vi "Decorate.vi"(8 "error in (no error)":errorcluster, 10 "Decorator":refnum<class "uPolicy.lvclass">, 11 "Decorate in":refnum<class "Decorate.lvclass">) -> (0 "error out":errorcluster, 3 "Decorate out":refnum<class "Decorate.lvclass">)   [LabVIEW 2023, in "uLib.lvlib" / "Decorate.lvclass"]
doc: "Append a subscription policy, expand the property node to append multiple policies."
uses:
  Decorate.lvclass
  uPolicy/uPolicy.lvclass
  Decorate.lvclass/Decorate.ctl
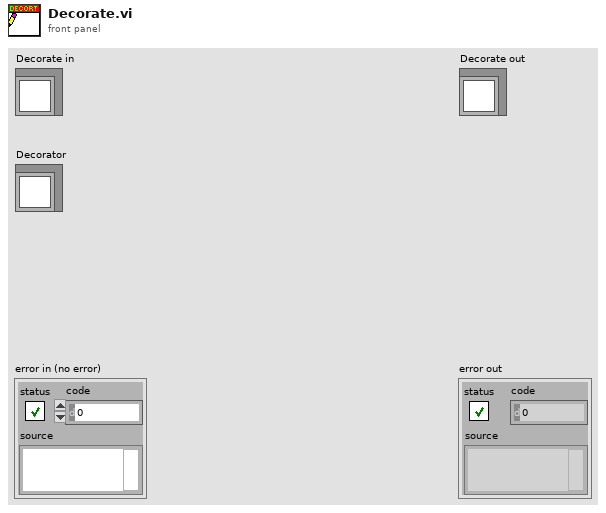
[diagram p1: front panel]
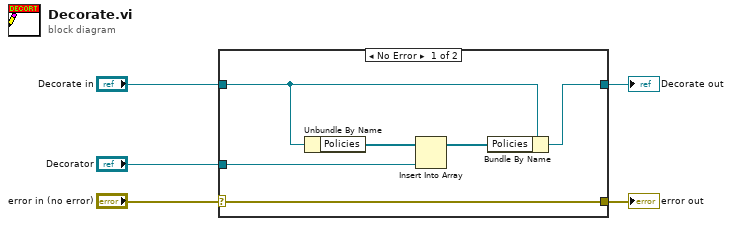
[diagram p0: block diagram]
diagram:
  n1 = case shown="No Error" "error in (no error)" {
    selector: "error in (no error)" -> [w11 w12]
    tunnel: [w11 w12] -> w4
    tunnel: [w10 w13] -> w2
    tunnel: "Decorate in" -> [w9 w13]
    tunnel: "Decorator" -> [w6 _]
    frame No Error {
      n2 = Unbundle By Name(w9) -> ("Policies"=w8:refnum<class "uPolicy.lvclass">[])
      n3 = Insert Into Array(array=w8, new element=w6) -> (w7:refnum<class "uPolicy.lvclass">[])  [unwired: 1 in]
      n4 = Bundle By Name(cluster=w9, "Policies"=w7) -> (w10:refnum<class "Decorate.lvclass">)
    }
    frame Error {
    }
  }
  "error out" <- w4
  "Decorate out" <- w2
